vi "Are All Objects Acquired.vi"(8 "error in (no error)":errorcluster, 11 "StorageService in":refnum<class "StorageService.lvclass">) -> (0 "error out":errorcluster, 2 "All Is Acquired?":bool, 3 "StorageService out":refnum<class "StorageService.lvclass">)   [LabVIEW 2014, in "StorageService.lvclass"]
uses:
  StorageService.lvclass
  StorageService.lvclass/StorageService.ctl
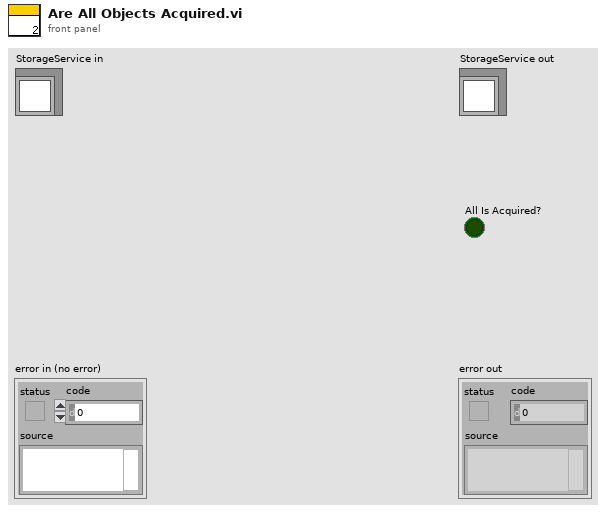
[diagram p1: front panel]
types:
  T1 = typedef "StorageService.lvclass/RegisteredObject.ctl" = cluster{"Name":string, "Is Acquired":bool, "Queue":refnum<queue>, "Message To Send":cluster{"Enqueuer":refnum<class "Message Enqueuer.lvclass">, "Message":refnum<class "ReplayData Msg.lvclass">}, "Save Parameters":variant}
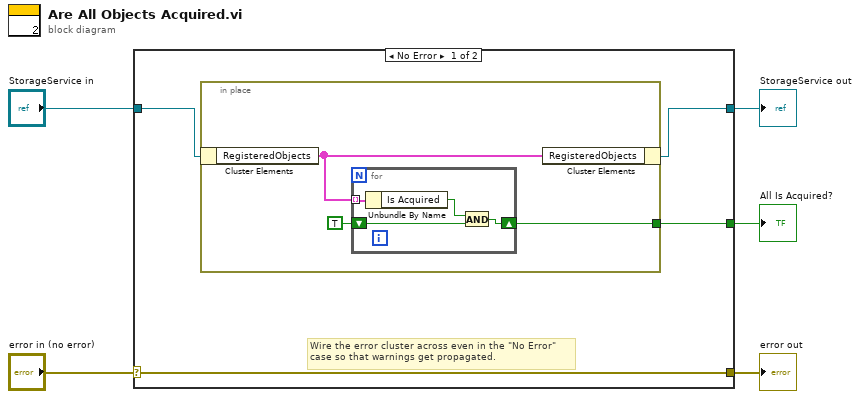
[diagram p0: block diagram]
diagram:
  n1 = case shown="No Error" "error in (no error)" {
    selector: "error in (no error)" -> [w9 w18]
    tunnel: [w9 w18] -> w4
    tunnel: [w7 w17] -> w2
    tunnel: "StorageService in" -> [w8 w17]
    tunnel: [w6 _] -> w1
    frame No Error {
      # "Wire the error cluster across even in the \"No Error\"\ncase so that warnings get propagated."
      n2 = in-place {
        in-place-border: [w10] -> w6
        n3 = in-place-cluster #1(w8) -> ("RegisteredObjects"=w11:T1[])
        n4 = for {
          tunnel: w11 -> [w16] mode=indexing
          shift-right: [w13] -> w10
          shift-left: TRUE -> [w14]
          n5 = Unbundle By Name(w16) -> ("Is Acquired"=w15:bool)
          n6 = And(x=w15, y=w14) -> (x .and. y?=w13:bool)
        }
        n7 = in-place-cluster #1("RegisteredObjects"=w11) -> (w7:refnum<class "StorageService.lvclass">)
      }
    }
    frame Error {
    }
  }
  "error out" <- w4
  "StorageService out" <- w2
  "All Is Acquired?" <- w1
